vi "Annotation_Read.vi"(8 "error in (no error)":errorcluster, 11 "Annotation Path (Source)":path=path "C:/Users/Admin/Desktop/Test Dataset/Annotations/vlcsnap-2023-06-05-13h54m01s380.txt") -> (0 "error out":errorcluster, 1 "Annotation Coords":sgl[][](array[numeric])=[[0.4479, 0.4583, 0.4583, 0.4694], [0.5109, 0.4611, 0.5198, 0.4713], [0.5089, 0.3815, 0.5177, 0.3907], [0.4807, 0.413, 0.4896, 0.4241], [0.4677, 0.3926, 0.4771, 0.4028], [0.4953, 0.2704, 0.5042, 0.2815]], 3 "Annotation Class":string[][](array[string])=[["Hit", "BBox"], ["Hit", "BBox"], ["Hit", "BBox"], ["Hit", "BBox"], ["Hit", "BBox"], ["Hit", "BBox"]])   [LabVIEW 2020]
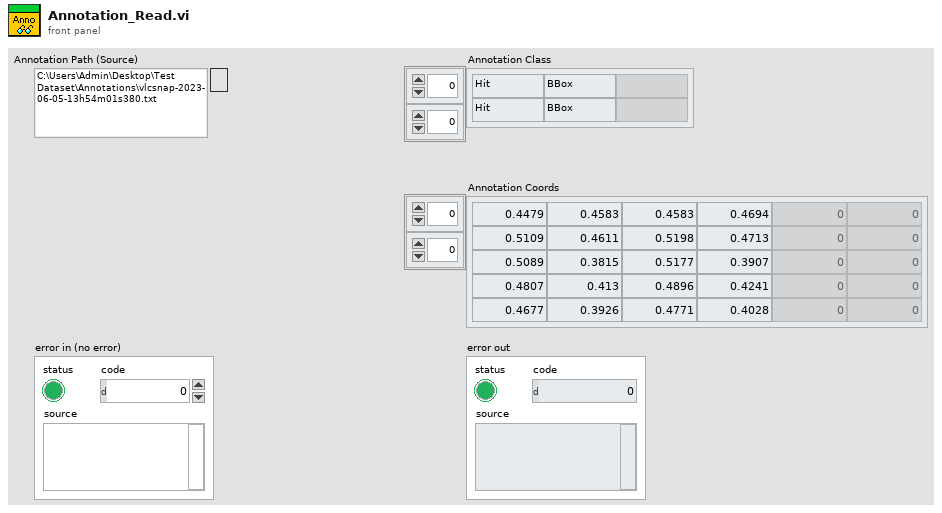
[diagram p1: front panel]
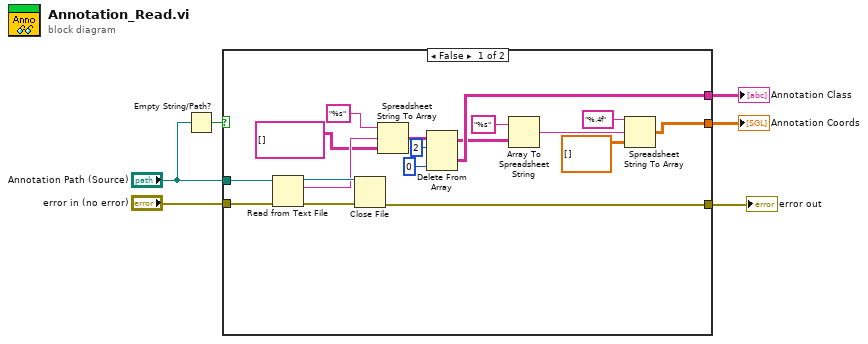
[diagram p0: block diagram]
diagram:
  n1 = Empty String/Path?(string/path="Annotation Path (Source)") -> (empty?=w1:bool)
  n2 = case shown="False" w1 {
    tunnel: [w24 w25] -> w6
    tunnel: "error in (no error)" -> [w22 w25]
    tunnel: "Annotation Path (Source)" -> [w21 _]
    tunnel: [w20 _] -> w4
    tunnel: [w19 _] -> w3
    frame False {
      n3 = Read from Text File(file (use dialog)=w21, error in=w22) -> (refnum out=w18:refnum<file>, text=w9:string, error out=w23:errorcluster)  [unwired: 2 in, 1 out]
      n4 = Close File(refnum=w18, error in=w23) -> (error out=w24:errorcluster)  [unwired: 1 out]
      n5 = Spreadsheet String To Array(format string="%s" ("format (%.3f)"), spreadsheet string=w9, array type (2D Dbl)=string[][] []) -> (array=w10:string[][])  [unwired: 1 in]
      n6 = Delete From Array(array=w10, length=2, index (col)=0 ("disabled index (col)")) -> (deleted portion=w19:string[][], array with subset deleted=w12:string[][])  [unwired: 1 in]
      n7 = Array To Spreadsheet String(array=w12, 3:"%s" ("format string")) -> (spreadsheet string=w14:string)  [unwired: 1 in]
      n8 = Spreadsheet String To Array(format string="%.4f" ("format (%.3f)"), spreadsheet string=w14, array type (2D Dbl)=sgl[][] []) -> (array=w20:sgl[][])  [unwired: 1 in]
    }
    frame True {
    }
  }
  "error out" <- w6
  "Annotation Coords" <- w4
  "Annotation Class" <- w3
